vi "Send Local Message_sushu.vi"(0 "Queue In":cluster{"Q":T1, "Name":string}, 1 "receiver process (\"\" - local)":string, 3 "Elements in Front":string, 5 "Elements at Back":string, 9 "message value":string, 11 "error in":errorcluster, 12 "message attributes":T2, 13 "timeout (-1 ms)":i32=-1) -> (4 "Queue Out":cluster{"Q":T1, "Name":string}, 10 "timed out?":bool, 15 "error out":errorcluster)   [LabVIEW 2021]
doc: "2015-02-03 15:04:39\n在同一个while循环内，可以使用多个字符串进行入队。\n在不同的while循环（例如在事件结构中）优先入队只限单个元素。\n多个元素时，必须在对胃入队。\nBug发现于2015-02-03，源于Gabe发现程序的一个Bug。\n蒋松\njiangsong@outlook.com\n\n基于AMC模块的二次封装，发送当个命令。\n20140304；\n\nAdds a message to the local message queue provided by the queue reference or to another message queue in the local application based on the receiver process name.\n\nIf \"priority message\" is True, the message will be added to the front of the message queue."
uses:
  <vilib>/NI/Tools/Keyed Array/KeyedArray.ctl
  <vilib>/NI/AMC/Message Queue.ctl
  <vilib>/NI/AMC/Message.ctl
  <vilib>/NI/AMC/Create Single Message.vi
  <vilib>/NI/AMC/Update Message Routing Info.vi
  <vilib>/NI/AMC/Send Message.vi
  <vilib>/NI/AMC/AMC.lvlib
  <vilib>/NI/Tools/Keyed Array/Tools_KeyedArray.lvlib
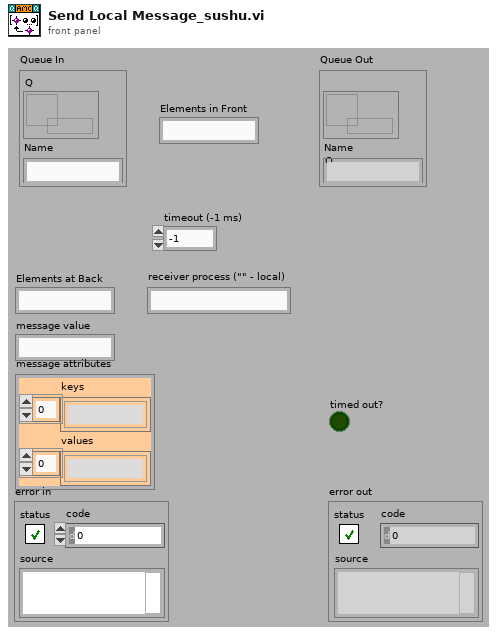
[diagram p1: front panel]
types:
  T1 = typedef "AMC.lvlib/Message Queue.ctl" = refnum<queue>
  T2 = typedef "Tools_KeyedArray.lvlib/KeyedArray.ctl" = cluster{"keys":string[], "values":string[]}
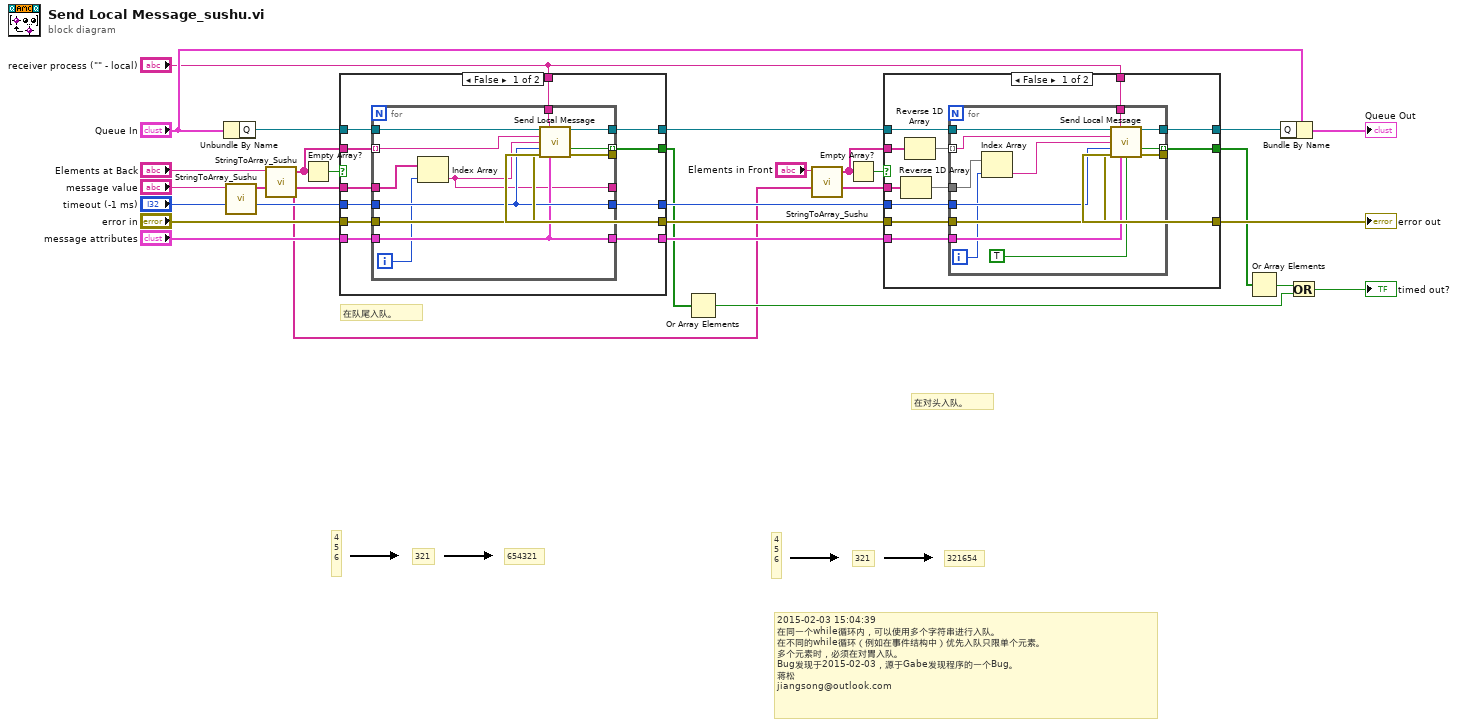
[diagram p0: block diagram]
diagram:
  # "2015-02-03 15:04:39\n在同一个while循环内，可以使用多个字符串进行入队。\n在不同的while循环（例如在事件结构中）优先入队只限单个元素。\n多个元素时，必须在对胃入队。\nBug发现于2015-02-03，源于Gabe发现程序的一个Bug。\n蒋松\njiangsong@outlook.com"
  # "321654"
  # "321"
  # "4\n5\n6"
  # "654321"
  # "321"
  # "4\n5\n6"
  # "在对头入队。"
  # "在队尾入队。"
  n1 = Unbundle By Name("Queue In") -> ("Q"=w23:T1)
  n2 = call <userlib>:"StringToArray_Sushu.vi"("State Queue"="message value") -> ("Array"=w1:string[])  [unwired: 7 in, 3 out]
  n3 = call <userlib>:"StringToArray_Sushu.vi"("State Queue"="Elements at Back") -> ("Array"=w22:string[])  [unwired: 7 in, 3 out]
  n4 = Empty Array?(array=w22) -> (empty?=w24:bool)
  n5 = case shown="False" w24 {
    tunnel: w23 -> [w38 w54]
    tunnel: "receiver process (\"\" - local)" -> [w37 _]
    tunnel: [w36 w54] -> w14
    tunnel: w1 -> [w35 _]
    tunnel: w22 -> [w34 _]
    tunnel: "error in" -> [w33 w53]
    tunnel: "timeout (-1 ms)" -> [w32 w52]
    tunnel: "message attributes" -> [w31 w51]
    tunnel: [w30 w53] -> w12
    tunnel: [w29 w52] -> w11
    tunnel: [w28 w51] -> w10
    tunnel: [w27 _] -> w7
    frame False {
      n6 = for {
        tunnel: w38 -> [w50]
        tunnel: w37 -> [w49]
        tunnel: [w48] -> w36
        tunnel: w34 -> [w47] mode=indexing
        tunnel: w35 -> [w43]
        tunnel: w33 -> [w46]
        tunnel: w32 -> [w42]
        tunnel: w31 -> [w41]
        tunnel: [w45] -> w27 mode=indexing
        tunnel: [w44] -> w30
        tunnel: [w40] -> _
        tunnel: [w42] -> w29
        tunnel: [w41] -> w28
        i -> [w39]
        n7 = Index Array(array=w43, index=w39) -> (element=w40:string)
        n8 = call <vilib>:"Send Local Message.vi"("message queue in"=w50, "receiver process (\"\" - local)"=w49, "message name"=w47, "message value"=w40, "timeout (-1 ms)"=w42, "error in"=w46, "message attributes"=w41) -> ("message queue out"=w48:T1, "timed out?"=w45:bool, "error out"=w44:errorcluster)  [unwired: 6 in]
      }
    }
    frame True {
    }
  }
  n9 = Or Array Elements(Boolean array=w7) -> (logical OR=w4:bool)
  n10 = call <userlib>:"StringToArray_Sushu.vi"("State Queue"="Elements in Front") -> ("Array"=w17:string[])  [unwired: 7 in, 3 out]
  n11 = Empty Array?(array=w17) -> (empty?=w16:bool)
  n12 = case shown="False" w16 {
    tunnel: w14 -> [w66 w81]
    tunnel: "receiver process (\"\" - local)" -> [w65 _]
    tunnel: [w64 w81] -> w9
    tunnel: w1 -> [w63 _]
    tunnel: w17 -> [w62 _]
    tunnel: w12 -> [w61 w80]
    tunnel: w11 -> [w60 _]
    tunnel: w10 -> [w59 _]
    tunnel: [w58 w80] -> w8
    tunnel: [w56 _] -> w6
    frame False {
      n13 = Reverse 1D Array(array=w63) -> (reversed array=w55:string[])
      n14 = Reverse 1D Array(array=w62) -> (reversed array=w57:string[])
      n15 = for {
        tunnel: w66 -> [w79]
        tunnel: w65 -> [w78]
        tunnel: [w77] -> w64
        tunnel: w57 -> [w76] mode=indexing
        tunnel: w55 -> [w75]
        tunnel: w61 -> [w74]
        tunnel: w60 -> [w73]
        tunnel: w59 -> [w72]
        tunnel: [w71] -> w56 mode=indexing
        tunnel: [w70] -> w58
        i -> [w67]
        n16 = Index Array(array=w75, index=w67) -> (element=w68:string)
        n17 = call <vilib>:"Send Local Message.vi"("message queue in"=w79, "receiver process (\"\" - local)"=w78, "message name"=w76, "message value"=w68, "timeout (-1 ms)"=w73, "error in"=w74, "message attributes"=w72, "priority message (F)"=TRUE) -> ("message queue out"=w77:T1, "timed out?"=w71:bool, "error out"=w70:errorcluster)  [unwired: 5 in]
      }
    }
    frame True {
    }
  }
  "error out" <- w8
  n18 = Or Array Elements(Boolean array=w6) -> (logical OR=w5:bool)
  n19 = Bundle By Name(cluster="Queue In", "Q"=w9) -> (→"Queue Out":cluster{"Q":T1, "Name":string})
  n20 = Or(x=w5, y=w4) -> (x .or. y?=→"timed out?":bool)
